vi "UI_Elmts_Refs[Labels].vi"(8 "error in (no error)":errorcluster, 10 "Elmts Labels":string[](array[string]), 11 "UI_Actor in":refnum<class "UI_Actor.lvclass">) -> (0 "error out":errorcluster, 1 "Founds":bool[](array[boolean]), 2 "Refs":refnum<vi>[](array[refnum]), 3 "UI_Actor out":refnum<class "UI_Actor.lvclass">)   [LabVIEW 2020, in "UI_Actor.lvlib" / "UI_Actor.lvclass"]
uses:
  UI_Actor.lvclass
  UI_Actor.lvclass/UI_Actor.ctl
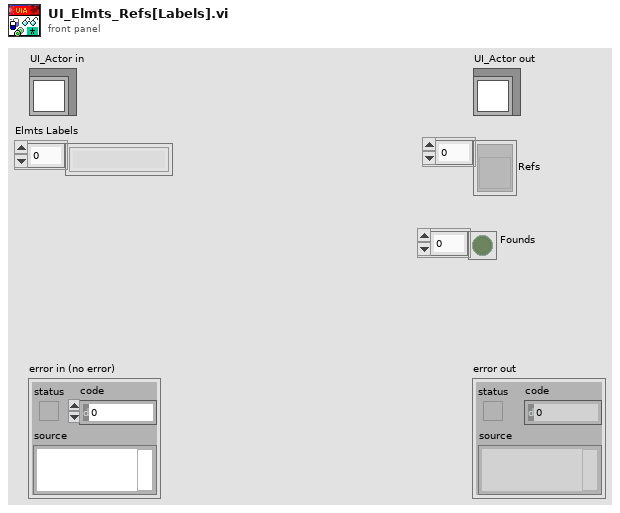
[diagram p1: front panel]
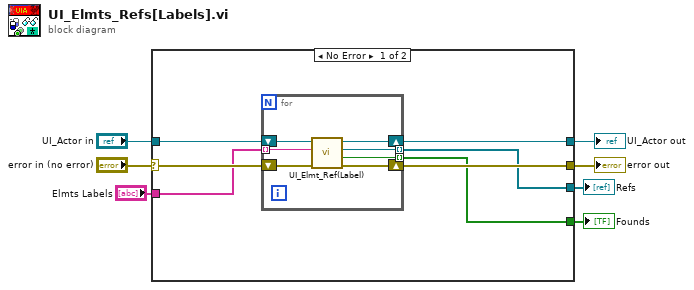
[diagram p0: block diagram]
diagram:
  n1 = case shown="No Error" "error in (no error)" {
    selector: "error in (no error)" -> [w12 w23]
    tunnel: [w11 w23] -> w6
    tunnel: [w13 w22] -> w4
    tunnel: "UI_Actor in" -> [w14 w22]
    tunnel: "Elmts Labels" -> [w10 _]
    tunnel: [w9 _] -> w1
    tunnel: [w8 _] -> w2
    frame No Error {
      n2 = for {
        shift-right: [w20] -> w13
        shift-left: w14 -> [w21]
        shift-right: [w18] -> w11
        shift-left: w12 -> [w19]
        tunnel: w10 -> [w17] mode=indexing
        tunnel: [w16] -> w9 mode=indexing
        tunnel: [w15] -> w8 mode=indexing
        n3 = call "UI_Elmt_Ref(Label).vi"("error in (no error)"=w19, "Elmt Label"=w17, "UI_Actor in"=w21) -> ("error out"=w18:errorcluster, "Found"=w15:bool, "Ctl Refnum"=w16:refnum<vi>, "UI_Actor out"=w20:refnum<class "UI_Actor.lvclass">)  [unwired: 5 in]
      }
    }
    frame Error {
    }
  }
  "error out" <- w6
  "UI_Actor out" <- w4
  "Founds" <- w2
  "Refs" <- w1
